vi "Write Byte order.vi"(8 "error in (no error)":errorcluster, 10 "Byte order":T1(ring)=enum."2-3-0-1", 11 "Protocol in":refnum<class "Protocol.lvclass">) -> (0 "error out":errorcluster, 3 "Protocol out":refnum<class "Protocol.lvclass">)   [LabVIEW 2016, in "Protocol.lvclass"]
uses:
  Protocol.lvclass
  Protocol.lvclass/Protocol.ctl
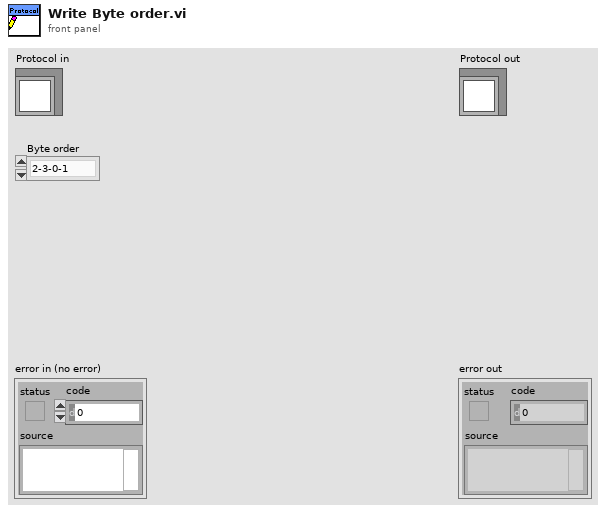
[diagram p1: front panel]
types:
  T1 = enum16{"0-1-2-3", "2-3-0-1", "1-0-3-2", "3-2-1-0"}
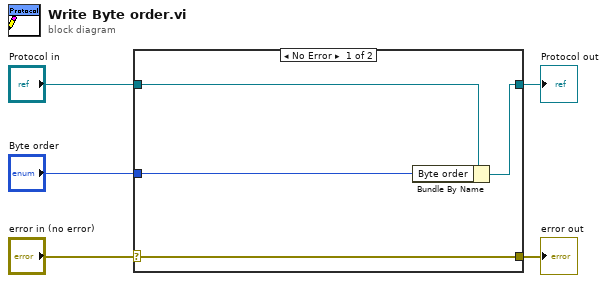
[diagram p0: block diagram]
diagram:
  n1 = case shown="No Error" "error in (no error)" {
    selector: "error in (no error)" -> [w9 w10]
    tunnel: [w9 w10] -> w4
    tunnel: [w7 w11] -> w2
    tunnel: "Protocol in" -> [w8 w11]
    tunnel: "Byte order" -> [w6 _]
    frame No Error {
      n2 = Bundle By Name(cluster=w8, "Byte order"=w6) -> (w7:refnum<class "Protocol.lvclass">)
    }
    frame Error {
    }
  }
  "error out" <- w4
  "Protocol out" <- w2
